vi "Auton Drive Dictation.vi"(8 "Reset Encoders":bool, 9 "Distance (inches)":dbl=52.0, 10 "Direction (0-359)":dbl, 11 "Speed (-1 to 1)":dbl=0.75) -> (0 "Joy Y":dbl=0.5124433303800191, 1 "Joy X":dbl, 2 "Distance Reached?":bool)   [LabVIEW 2014]
uses:
  Begin/Global RefNums.vi
  <vilib>/addons/control/pid/NI_PID_pid.lvlib
  <vilib>/addons/control/pid/pid.llb/PID (DBL).vi
panel:
  in  "y":dbl=3.0
  in  "Sigma Conversion":dbl=4.0 format="%#_13g"
  in  "output range":cluster{"output high":dbl, "output low":dbl}={"output high"=1.0, "output low"=-1.0} {"output low" format="%.2f"; "output high" format="%.2f"}
  out "Counts":i32=337
  in  "PID Range":dbl=50.0 format="%#_13g"
  in  "PID gains":T1={"proportional gain (Kc)"=0.01, "integral time (Ti, min)"=0.0, "derivative time (Td, min)"=0.0} {"derivative time (Td, min)" format="%.3f"; "integral time (Ti, min)" format="%.7f"; "proportional gain (Kc)" format="%.3f"}
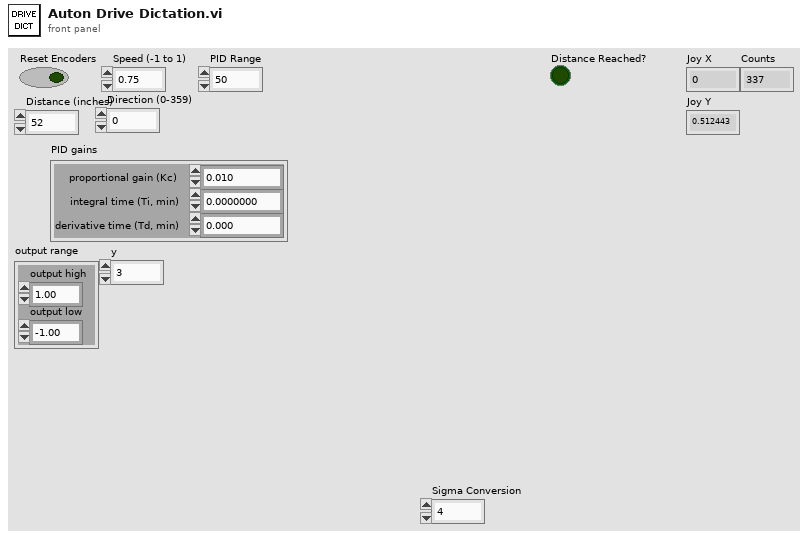
[diagram p1: front panel]
types:
  T1 = cluster{"proportional gain (Kc)":dbl, "integral time (Ti, min)":dbl, "derivative time (Td, min)":dbl}
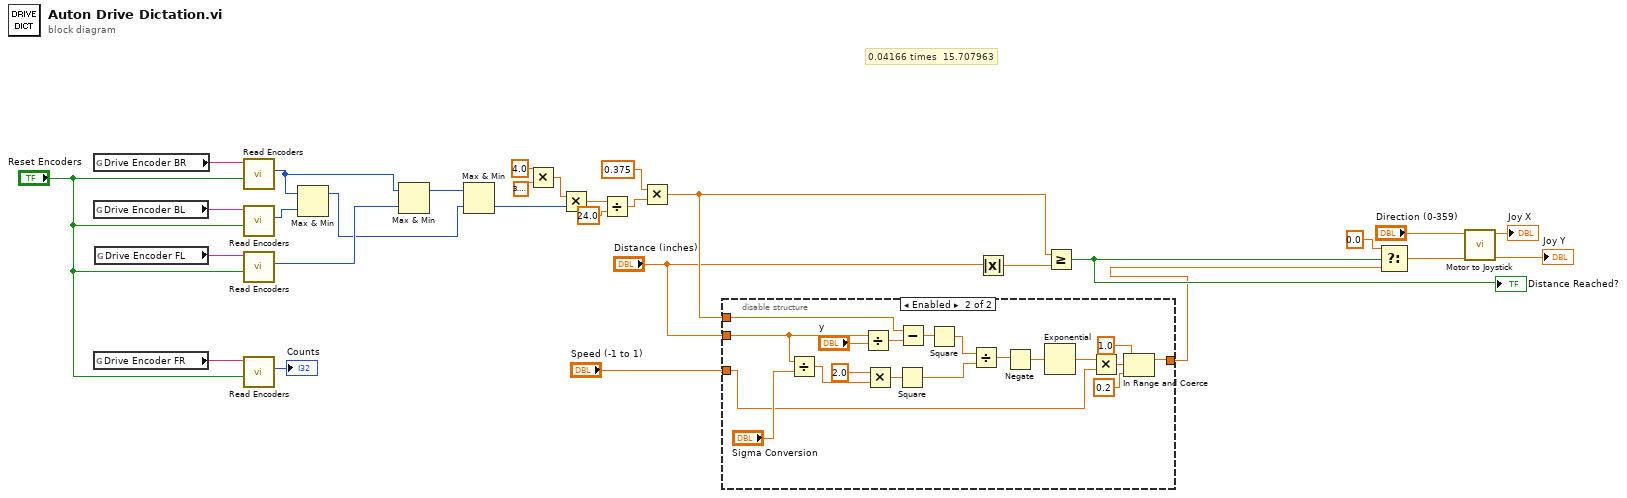
[diagram p0: block diagram]
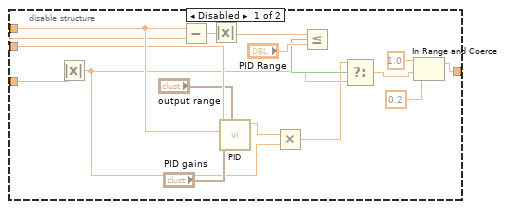
[diagram p2: hidden frame]
diagram:
  # "0.04166 times  15.707963"
  n1 = global read "Global RefNums.vi" "Drive Encoder BR"() -> (w30:string)
  n2 = global read "Global RefNums.vi" "Drive Encoder BL"() -> (w16:string)
  n3 = global read "Global RefNums.vi" "Drive Encoder FR"() -> (w11:string)
  n4 = global read "Global RefNums.vi" "Drive Encoder FL"() -> (w14:string)
  n5 = call "Read Encoders.vi"("Reset Encoders"="Reset Encoders", "Encoder"=w30) -> ("Counts"=w8:i32)  [unwired: 9 in]
  n6 = call "Read Encoders.vi"("Reset Encoders"="Reset Encoders", "Encoder"=w16) -> ("Counts"=w15:i32)  [unwired: 9 in]
  n7 = call "Read Encoders.vi"("Reset Encoders"="Reset Encoders", "Encoder"=w14) -> ("Counts"=w7:i32)  [unwired: 9 in]
  n8 = call "Read Encoders.vi"("Reset Encoders"="Reset Encoders", "Encoder"=w11) -> ("Counts"=→"Counts":i32)  [unwired: 9 in]
  n9 = Max & Min(x=w8, y=w15) -> (max(x,y)=w5:i32)  [unwired: 1 out]
  n10 = Max & Min(x=w8, y=w7) -> (max(x,y)=w6:i32)  [unwired: 1 out]
  n11 = Max & Min(x=w6, y=w5) -> (min(x,y)=w4:i32)  [unwired: 1 out]
  n12 = Multiply(x=4.0, y=3.141592653589793) -> (x*y=w23:dbl)
  n13 = Multiply(x=w23, y=w4) -> (x*y=w22:dbl)
  n14 = Divide(x=w22, y=24.0) -> (x/y=w21:dbl)
  n15 = Multiply(x=0.375 ("y"), y=w21) -> (x*y=w19:dbl)
  n16 = disable-structure shown="Enabled" {
    disable-tunnel: w19 -> [w43 w48]
    disable-tunnel: "Distance (inches)" -> [w40 w49]
    disable-tunnel: "Speed (-1 to 1)" -> [w38 w50]
    disable-tunnel: [w31 w51] -> w2
    frame Disabled {
      n17 = Absolute Value(x=w38) -> (abs(x)=w37:dbl)
      n18 = Subtract(x=w43, y=w40) -> (x-y=w45:dbl)
      n19 = Absolute Value(x=w45) -> (abs(x)=w44:dbl)
      n20 = call-poly <vilib>:"PID.vi"("output range"="output range", "PID gains"="PID gains", "process variable"=w43, "setpoint"=w40) -> ("output"=w36:dbl)  [unwired: 6 in, 1 out]
      n21 = Multiply(x=w36, y=w37) -> (x*y=w35:dbl)
      n22 = Less Or Equal?(x=w44, y="PID Range") -> (x <= y?=w41:bool)
      n23 = Select(t=w35, s=w41, f=w37) -> (s? t:f=w32:dbl)
      n24 = In Range and Coerce(upper limit=1.0, x=w32, lower limit=0.2) -> (coerced(x)=w31:dbl)  [unwired: 1 out]
    }
    frame Enabled {
      n25 = Divide(x=w49, y="Sigma Conversion") -> (x/y=w55:dbl)
      n26 = Divide(x=w49, y="y") -> (x/y=w65:dbl)
      n27 = Multiply(x=2.0 ("y"), y=w55) -> (x*y=w62:dbl)
      n28 = Square(x=w62) -> (x^2=w61:dbl)
      n29 = Subtract(x=w48, y=w65) -> (x-y=w64:dbl)
      n30 = Square(x=w64) -> (x^2=w60:dbl)
      n31 = Divide(x=w60, y=w61) -> (x/y=w59:dbl)
      n32 = Negate(x=w59) -> (-x=w58:dbl)
      n33 = Exponential(1:w58) -> (0:w57:dbl)
      n34 = Multiply(x=w57, y=w50) -> (x*y=w54:dbl)
      n35 = In Range and Coerce(upper limit=1.0, x=w54, lower limit=0.2) -> (coerced(x)=w51:dbl)  [unwired: 1 out]
    }
  }
  n36 = Absolute Value(x="Distance (inches)") -> (abs(x)=w17:dbl)
  n37 = Greater Or Equal?(x=w19, y=w17) -> (x >= y?=w29:bool)
  "Distance Reached?" <- w29
  n38 = Select(t=0.0, s=w29, f=w2) -> (s? t:f=w27:dbl)
  n39 = call "Motor to Joystick.vi"("Drive Motor"=w27, "Rotational Motor"="Direction (0-359)") -> ("Joy Y"=→"Joy Y":dbl, "Joy X"=→"Joy X":dbl)  [unwired: 8 in]
